vi "CheckParameters.vi"(8 "error in (no error)":errorcluster, 10 "Parameters":u32[](array[numeric]), 11 "Spannungseinbruch in":refnum<class "Spannungseinbruch.lvclass">) -> (0 "error out":errorcluster, 3 "Spannungseinbruch out":refnum<class "Spannungseinbruch.lvclass">)   [LabVIEW 2013, in "Spannungseinbruch.lvclass"]
uses:
  Spannungseinbruch.lvclass
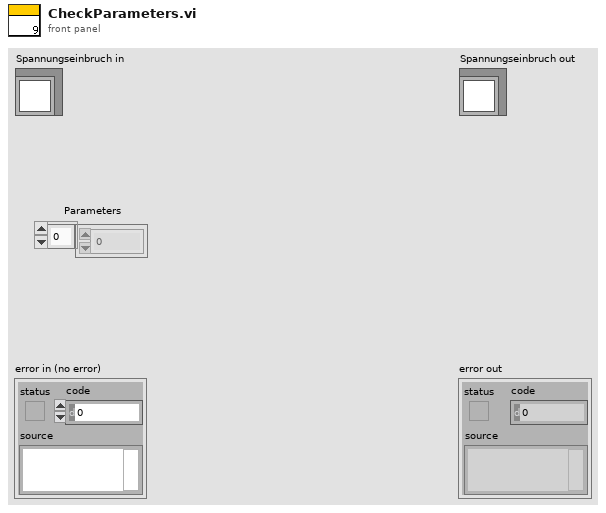
[diagram p1: front panel]
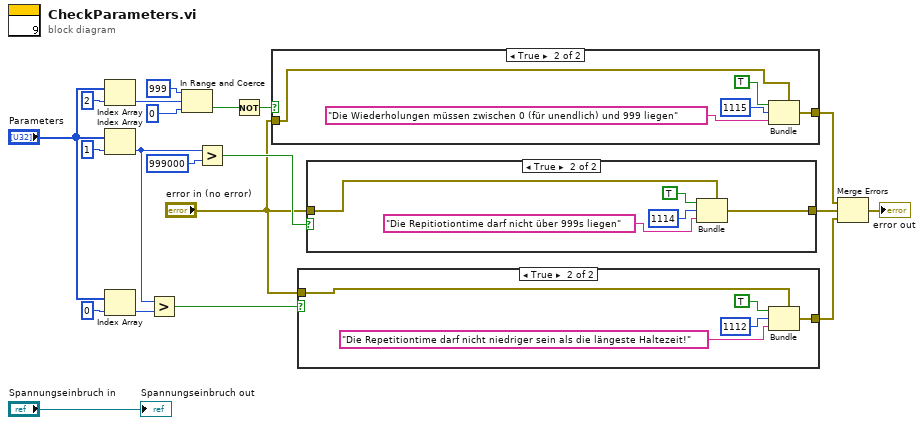
[diagram p0: block diagram]
diagram:
  n1 = Index Array(array="Parameters", index=2) -> (element=w7:u32)
  n2 = Index Array(array="Parameters", index=1) -> (element=w2:u32)
  n3 = Index Array(array="Parameters", index=0) -> (element=w1:u32)
  n4 = Greater?(x=w2, y=w1) -> (0:w17:bool)
  n5 = In Range and Coerce(upper limit=u32 999, x=w7, lower limit=u32 0) -> (In Range?=w6:bool)  [unwired: 1 out]
  n6 = Greater?(x=w2, y=u32 999000) -> (0:w10:bool)
  n7 = Not(x=w6) -> (.not. x?=w5:bool)
  n8 = case shown="True" w5 {
    tunnel: [w21 w23] -> w3
    tunnel: "error in (no error)" -> [w21 w22]
    frame False {
    }
    frame True {
      n9 = Bundle(cluster=w22, "status"=TRUE, "code"=1115, "source"="Die Wiederholungen müssen zwischen 0 (für unendlich) und 999 liegen") -> (w23:errorcluster)
    }
  }
  n10 = case shown="True" w17 {
    tunnel: "error in (no error)" -> [w27 w32]
    tunnel: [w27 w28] -> w16
    frame False {
    }
    frame True {
      n11 = Bundle(cluster=w32, "status"=TRUE, "code"=1112, "source"="Die Repetitiontime darf nicht niedriger sein als die längeste Haltezeit!") -> (w28:errorcluster)
    }
  }
  n12 = case shown="True" w10 {
    tunnel: "error in (no error)" -> [w33 w38]
    tunnel: [w33 w34] -> w11
    frame False {
    }
    frame True {
      n13 = Bundle(cluster=w38, "status"=TRUE, "code"=1114, "source"="Die Repitiotiontime darf nicht über 999s liegen") -> (w34:errorcluster)
    }
  }
  n14 = Merge Errors(w3, w11, w16) -> (→"error out":errorcluster)
  "Spannungseinbruch out" <- "Spannungseinbruch in"
